vi "SDO download (U32).vi"(6 "Value":u32, 7 "Wait?":bool, 8 "error in (no error)":errorcluster, 9 "Multiplexor":T1 {"Index" format="%04x"}, 10 "Node ID":u8, 11 "CANopen in":refnum<class "CANopen.lvclass">) -> (0 "error out":errorcluster, 3 "CANopen out":refnum<class "CANopen.lvclass">)   [LabVIEW 2024, in "canopen.lvlib" / "CANopen.lvclass"]
doc: "Writes a value in the open dictionary of a CANopen node."
uses:
  CANopen.lvclass
  CANopen.lvclass/CANopen.ctl
  Multiplexor.ctl
  CANopen Master.lvlib
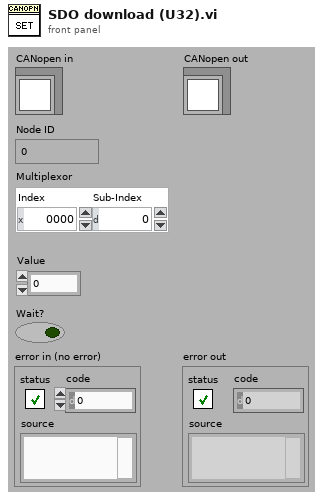
[diagram p1: front panel]
types:
  T1 = typedef "CANopen Master.lvlib/Multiplexor.ctl" = cluster{"Index":u16, "Sub-Index":u8}
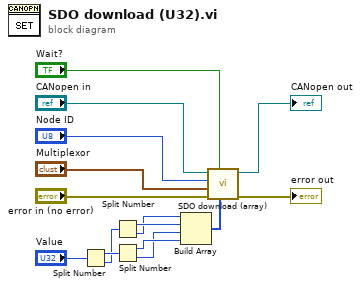
[diagram p0: block diagram]
diagram:
  n1 = Split Number(x="Value") -> (hi(x)=w3:u16, lo(x)=w2:u16)
  n2 = Split Number(x=w2) -> (hi(x)=w7:u8, lo(x)=w6:u8)
  n3 = Split Number(x=w3) -> (hi(x)=w5:u8, lo(x)=w4:u8)
  n4 = Build Array(w6, w7, w4, w5) -> (w9:u8[])
  n5 = call "SDO download (array).vi"("Value"=w9, "Wait?"="Wait?", "error in"="error in (no error)", "Multiplexor"="Multiplexor", "Node ID"="Node ID", "CANopen in"="CANopen in") -> ("error out"=→"error out":errorcluster, "CANopen out"=→"CANopen out":refnum<class "CANopen.lvclass">)  [unwired: 4 in]
